vi "QuantileTransformer.vi"(8 "error in (no error)":errorcluster caption="entrée d'erreur (pas d'erreur)", 11 "QuantileTransformer":T1={"n_quantiles"=1000, "output_distribution"="uniform", "ignore_implicit_zeros"=FALSE, "subsample"=100000.0, "random_state"=-1, "copy"=TRUE} {"random_state" min=-1}) -> (0 "error out":errorcluster, 3 "QuantileTransformer.lvclass":refnum<class "QuantileTransformer.lvclass">)   [LabVIEW 2020]
doc: "Transform features using quantiles information.\n\nThis method transforms the features to follow a uniform or a normal distribution. Therefore, for a given feature, this transformation tends to spread out the most frequent values. It also reduces the impact of (marginal) outliers: this is therefore a robust preprocessing scheme.\n\nThe transformation is applied on each feature independently. First an estimate of the cumulative distribution function of a feature is used to map the original values to a uniform distribution. The obtained values are then mapped to the desired output distribution using the associated quantile function. Features values of new/unseen data that fall below or above the fitted range will be mapped to the bounds of the output distribution. Note that this transform is non-linear. It may distort linear correlations between variables measured at the same scale but renders variables measured at different scales more directly comparable.\n\n\nParameters : \n\n- n_quantiles : int, optional (default=1000 or n_samples)\nNumber of quantiles to be computed. It corresponds to the number of landmarks used to discretize the cumulative distribution function. If n_quantiles is larger than the number of samples, n_quantiles is set to the number of samples as a larger number of quantiles does not give a better approximation of the cumulative distribution function estimator.\n\n- output_distribution : str, optional (default=’uniform’)\nMarginal distribution for the transformed data. The choices are ‘uniform’ (default) or ‘normal’.\n\n- ignore_implicit_zeros : bool, optional (default=False)\nOnly applies to sparse matrices. If True, the sparse entries of the matrix are discarded to compute the quantile statistics. If False, these entries are treated as zeros.\n\n- subsample : int, optional (default=1e5)\nMaximum number of samples used to estimate the quantiles for computational efficiency. Note that the subsampling procedure may differ for value-identical sparse and dense matrices.\n\n- random_state : int, RandomState instance or None, optional (default=None=-1)\nDetermines random number generation for subsampling and smoothing noise. Please see subsample for more details. Pass an int for reproducible results across multiple function calls. \n\n- copy : boolean, optional, (default=True)\nSet to False to perform inplace transformation and avoid a copy (if the input is already a numpy array).\n\n\n\nMethods :\n\n\n- Fit : Compute the quantiles used for transforming.\n\nParameters : \n\nX : ndarray or sparse matrix, shape (n_samples, n_features)\nThe data used to scale along the features axis. If a sparse matrix is provided, it will be converted into a sparse csc_matrix. Additionally, the sparse matrix needs to be nonnegative if ignore_implicit_zeros\n\n\n- Fit Transform : Fit to data, then transform it. Fits transformer to X and y with optional parameters fit_params and returns a transformed version of X.\n\nParameters :\n\nX : {array-like, sparse matrix, dataframe} of shape (n_samples, n_features)\n\ny : ndarray of shape (n_samples,), default=None\nTarget values..\n\nReturns : \n\nX_new : ndarray array of shape (n_samples, n_features_new)\nTransformed array.\n\n\n- Transform : Feature-wise transformation of the data.\n\nParameters : \n\nX : ndarray or sparse matrix, shape (n_samples, n_features)\nThe data used to scale along the features axis. If a sparse matrix is provided, it will be converted into a sparse csc_matrix. Additionally, the sparse matrix needs to be nonnegative if ignore_implicit_zeros is False.\n\nReturns : \n\nXt : ndarray or sparse matrix, shape (n_samples, n_features)\nThe projected data."
uses:
  QuantileTransformer.lvclass
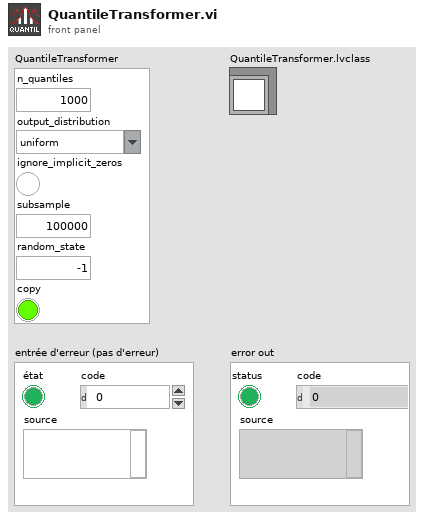
[diagram p1: front panel]
types:
  T1 = cluster{"n_quantiles":i32, "output_distribution":string, "ignore_implicit_zeros":bool, "subsample":dbl, "random_state":i32, "copy":bool}
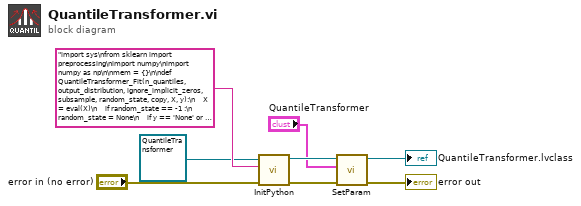
[diagram p0: block diagram]
diagram:
  n1 = call-dynamic "InitPython.vi"("error in (no error)"="error in (no error)", "Python Instruction"="import sys\nfrom sklearn import preprocessing\nimport numpy\nimport numpy as np\n\nmem = {}\n\ndef QuantileTransformer_Fit(n_quantiles, output_distribution, ignore_implicit_zeros, subsample, random_state, copy, X, y):\n    X = eval(X)\n    if random_state == -1 :\n        random_state = None\n    if y == 'None' or y == '':\n        y = None\n    else:\n        y = eval(y)\n    try:\n        QuantileTransformer = preprocessing.QuantileTransformer(n_quantiles, output_distribution, ignore_implicit_zeros, subsample, random_state, copy).fit(X, y)\n        mem['FitQuantileTransformer'] = QuantileTransformer\n        return str('OK')\n    except:\n        erreur = sys.exc_info()\n        typerr = u\"%s\" % (erreur[0])\n        typerr = typerr[typerr.find(\"'\")+1:typerr.rfind(\"'\")]\n        msgerr = u\"%s\" % (erreur[1])\n        message = str('/!\\\\ {0} : {1}'. format(typerr,msgerr))\n        return message \n    \ndef QuantileTransformer_FitTransform(n_quantiles, output_distribution, ignore_implicit_zeros, subsample, random_state, copy, X, y):\n    X = eval(X)\n    if random_state == -1 :\n        random_state = None\n    if y == 'None' or y == '':\n        y = None\n    else:\n        y = eval(y)\n    try:\n        QuantileTransformer = preprocessing.QuantileTransformer(n_quantiles, output_distribution, ignore_implicit_zeros, subsample, random_state, copy).fit_transform(X, y)\n        dtype = type(QuantileTransformer)\n        if dtype == numpy.ndarray:\n            QuantileTransformer = QuantileTransformer.tolist()\n            return str(QuantileTransformer) \n        else:\n            Mat = QuantileTransformer.tocoo()\n            return str(list(zip(Mat.row, Mat.col, Mat.data)))\n    except:\n        erreur = sys.exc_info()\n        typerr = u\"%s\" % (erreur[0])\n        typerr = typerr[typerr.find(\"'\")+1:typerr.rfind(\"'\")]\n        msgerr = u\"%s\" % (erreur[1])\n        message = str('/!\\\\ {0} : {1}'. format(typerr,msgerr))\n        return message \n\ndef QuantileTransformer_Transform(n_quantiles, output_distribution, ignore_implicit_zeros, subsample, random_state, copy, X, y):\n    X = eval(X)\n    if random_state == -1 :\n        random_state = None\n    if y == 'None' or y == '':\n        y = None\n    else:\n        y = eval(y)\n    try:\n        QuantileTransformer = mem['FitQuantileTransformer'].transform(X)\n        dtype = type(QuantileTransformer)\n        if dtype == numpy.ndarray:\n            QuantileTransformer = QuantileTransformer.tolist()\n            return str(QuantileTransformer) \n        else:\n            Mat = QuantileTransformer.tocoo()\n            return str(list(zip(Mat.row, Mat.col, Mat.data)))\n    except:\n        erreur = sys.exc_info()\n        typerr = u\"%s\" % (erreur[0])\n        typerr = typerr[typerr.find(\"'\")+1:typerr.rfind(\"'\")]\n        msgerr = u\"%s\" % (erreur[1])\n        message = str('/!\\\\ {0} : {1}'. format(typerr,msgerr))\n        return message", "Scikit-learn en entrée"=refnum<class "QuantileTransformer.lvclass"> refnum ("QuantileTransformer.lvclass")) -> ("error out"=w4:errorcluster, "Scikit-learn en sortie"=w5:refnum<class "QuantileTransformer.lvclass">)  [unwired: 7 in]
  n2 = call-dynamic "SetParam.vi"("error in (no error)"=w4, "QuantileTransformer"="QuantileTransformer", "QuantileTransformer.lvclass"=w5) -> ("error out"=→"error out":errorcluster, "QuantileTransformer.lvclass"=→"QuantileTransformer.lvclass":refnum<class "QuantileTransformer.lvclass">)  [unwired: 7 in]
